vi "RW Storage Test.vi"() -> (0 "error out":errorcluster, 2 "Pass":bool)   [LabVIEW 2021]
uses:
  typedef/Query Keys Return.ctl
  typedef/Zenoh Configuration.ctl
  Zenoh.lvclass/Zenoh.ctl
  Wrappers/Put Raw Wrapper.vi
  Core/Write Double.vi/58400e5e-2cc1-4aca-8f0f-3a78c0a2476e.vi
  Wrappers/Query Keys Wrapper.vi
  Wrappers/Poll Raw Wrapper.vi
  Core/Read Double.vi/4c4e9aed-29a9-49a4-ae79-bb096e87db4b.vi
  SubVIs/Get Zenoh Path.vi
  Core/Write Double.vi/58400e5e-2cc1-4aca-8f0f-3a78c0a2476e.vi/c28b0ead-42ad-4072-80a2-aca7f2bd7ce3.vi
  Core/Write Double.vi/58400e5e-2cc1-4aca-8f0f-3a78c0a2476e.vi/d83f0d1e-b5f2-409c-a855-55c666a7c55e.vi
  Core/Write Double.vi/58400e5e-2cc1-4aca-8f0f-3a78c0a2476e.vi/e02991d1-a06a-4e5e-a573-6dce97b92612.vi
  SubVIs/Add Zenoh Error.vi
  Core/Read Double.vi/4c4e9aed-29a9-49a4-ae79-bb096e87db4b.vi/c28b0ead-42ad-4072-80a2-aca7f2bd7ce3.vi
  Core/Read Double.vi/4c4e9aed-29a9-49a4-ae79-bb096e87db4b.vi/48104490-ec73-4168-8754-ff252ec03617.vi
  <vilib>/CIF Foundation/CIF Utilities/DataTypes/SubVIs/DataTypes Error.vi
  Core/Read Double.vi/4c4e9aed-29a9-49a4-ae79-bb096e87db4b.vi/543c0f61-77eb-4f29-b175-1688c1700ba4.vi
  <vilib>/CIF Foundation/CIF Utilities/DataTypes/SubVIs/DataTypes Error Core.vi
  SubVIs/Add Zenoh Error Core.vi
  Zenoh.lvclass
panel:
  out "Query Key Return":T1 {"Data Bytes" format="%.0x"; "Key Bytes" format="%.0x"}
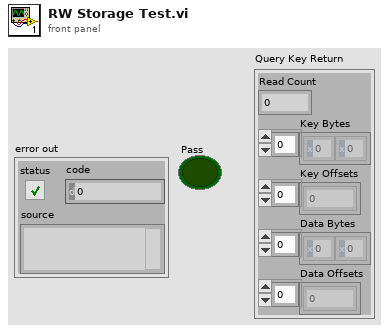
[diagram p1: front panel]
types:
  T1 = typedef "Zenoh.lvclass/Query Keys Return.ctl" = cluster{"Read Count":i32, "Key Bytes":u8[], "Key Offsets":u32[], "Data Bytes":u8[], "Data Offsets":u32[]}
  T2 = typedef "Zenoh.lvclass/Zenoh Configuration.ctl" = cluster{"Configuration (file or JSON)":string, "Liveliness":bool, "Liveliness Name":string, "Storage Key Expressions":string[]}
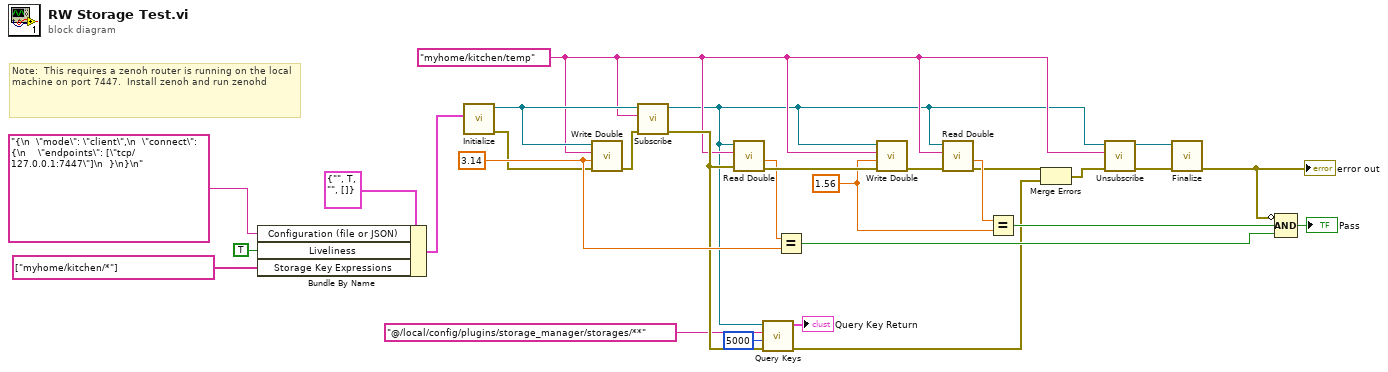
[diagram p0: block diagram]
diagram:
  w22 = 1.56 ("Numeric")
  w24 = 3.14 ("Numeric")
  w6 = "myhome/kitchen/temp" ("key")
  # "Note:  This requires a zenoh router is running on the local machine on port 7447.  Install zenoh and run zenohd"
  n1 = Bundle By Name(cluster=T2 {"Configuration (file or JSON)"="", "Liveliness"=TRUE, "Liveliness Name"="", "Storage Key Expressions"=[]} ("Zenoh Configuration"), "Configuration (file or JSON)"="{\n  \"mode\": \"client\",\n  \"connect\": {\n    \"endpoints\": [\"tcp/127.0.0.1:7447\"]\n  }\n}\n" ("value"), "Liveliness"=TRUE, "Storage Key Expressions"=string[] ["myhome/kitchen/*"]) -> (w10:T2)
  n2 = call "Initialize.vi"("Zenoh Configuration"=w10) -> ("error out"=w16:errorcluster, "Zenoh out"=w17:refnum<class "Zenoh.lvclass">)  [unwired: 9 in]
  n3 = call "Write Double.vi"("error in (no error)"=w16, "Numeric"=w24, "Key"=w6, "Zenoh in"=w17) -> ("error out"=w15:errorcluster)  [unwired: 7 in]
  n4 = call "Subscribe.vi"("error in (no error)"=w15, "Key"=w6, "Zenoh in"=w17) -> ("error out"=w14:errorcluster, "Zenoh out"=w5:refnum<class "Zenoh.lvclass">)  [unwired: 7 in]
  n5 = call "Read Double.vi"("error in (no error)"=w14, "Key"=w6, "Zenoh in"=w5) -> ("error out"=w29:errorcluster, "Numeric Out"=w25:dbl)  [unwired: 6 in, 1 out]
  n6 = call "Query Keys.vi"("error in (no error)"=w14, "timeout_ms"=u64 5000, "Query Expression"="@/local/config/plugins/storage_manager/storages/**", "Zenoh in"=w5) -> ("error out"=w3:errorcluster, "Query Key Return"=→"Query Key Return":T1)  [unwired: 6 in]
  n7 = Equal?(x=w25, y=w24) -> (x = y?=w21:bool)
  n8 = call "Write Double.vi"("error in (no error)"=w29, "Numeric"=w22, "Key"=w6, "Zenoh in"=w5) -> ("error out"=w28:errorcluster)  [unwired: 7 in]
  n9 = call "Read Double.vi"("error in (no error)"=w28, "Key"=w6, "Zenoh in"=w5) -> ("error out"=w4:errorcluster, "Numeric Out"=w23:dbl)  [unwired: 6 in, 1 out]
  n10 = Equal?(x=w23, y=w22) -> (x = y?=w20:bool)
  n11 = Merge Errors(w4, w3) -> (w2:errorcluster)
  n12 = call "Unsubscribe.vi"("error in (no error)"=w2, "Key"=w6, "Zenoh in"=w5) -> ("error out"=w27:errorcluster, "Zenoh out"=w26:refnum<class "Zenoh.lvclass">)  [unwired: 7 in]
  n13 = call "Finalize.vi"("error in (no error)"=w27, "Zenoh in"=w26) -> ("error out"=w19:errorcluster)  [unwired: 8 in, 1 out]
  "error out" <- w19
  n14 = Compound Arithmetic op=AND(invert w19, w20, w21) -> (→"Pass":bool)
